vi "Removable devices detection v8.5.vi"() -> (0 "Drive Number":i32, 1 "Drives":string[](array[string]), 2 "Drives Types":T1(array[ring]), 3 "Removable":bool, 4 "Removable":string[](array[string]))   [LabVIEW 2016, in "斯坦道CODMn.lvlib"]
uses:
  kernel32.dll
panel:
  out "Count":i32
  in  "stop":bool
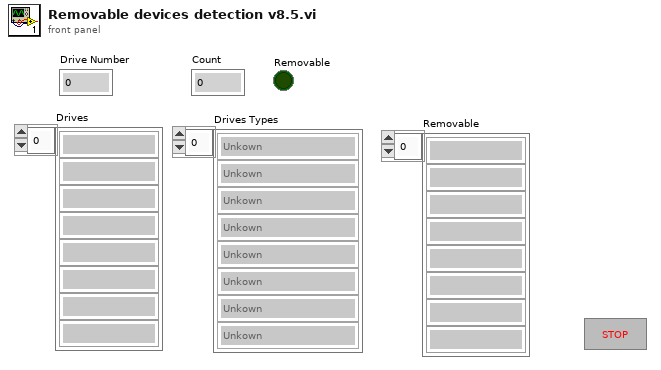
[diagram p1: front panel]
types:
  T1 = enum16{"Unkown", "No Root", "Removable", "Fixed", "Remote Drive", "CD Rom", "Ramdisk"}[]
  T2 = enum16{"Unkown", "No Root", "Removable", "Fixed", "Remote Drive", "CD Rom", "Ramdisk"}
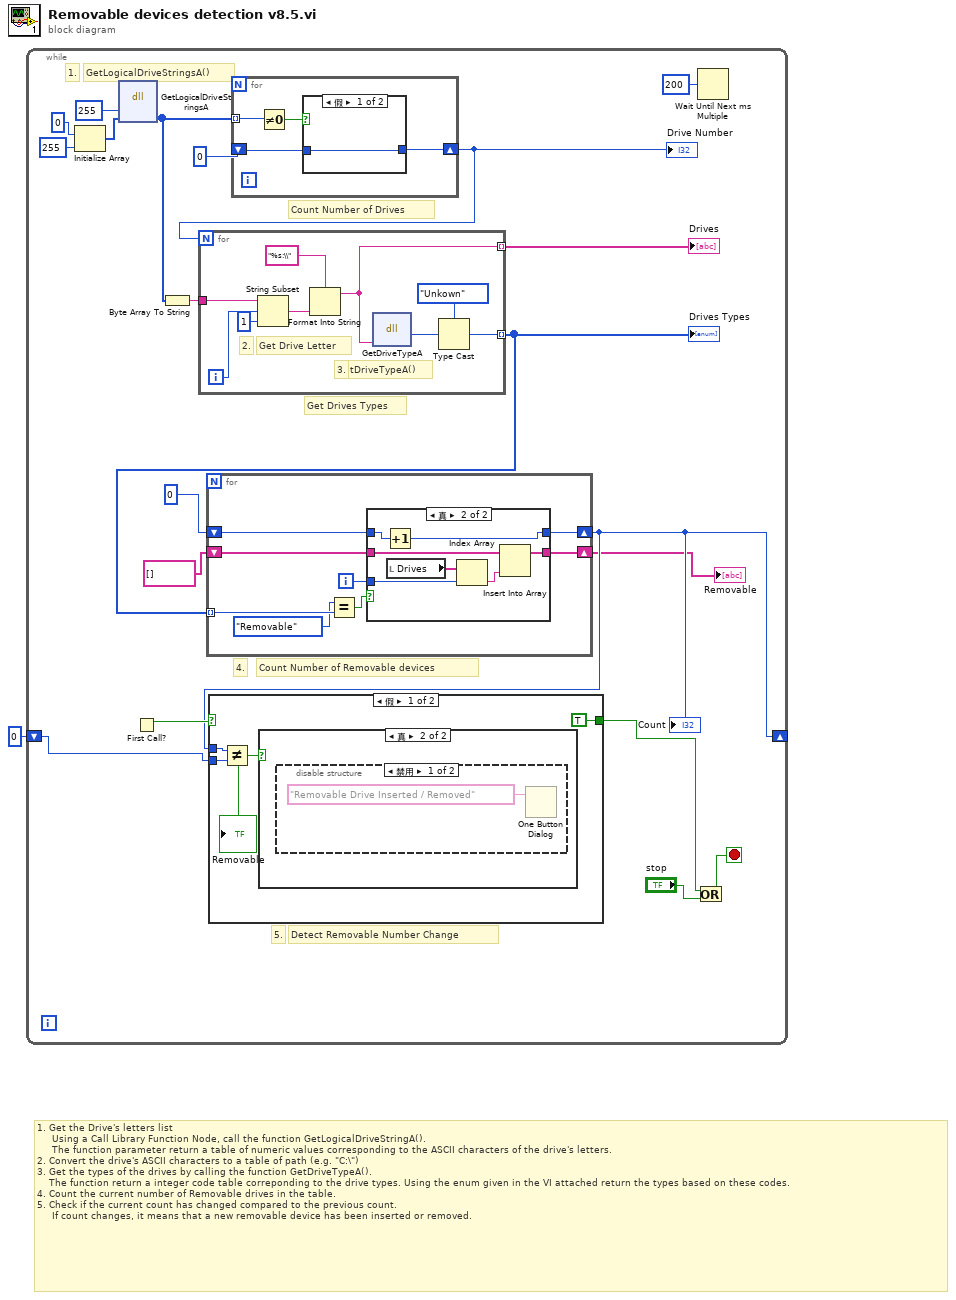
[diagram p0: block diagram]
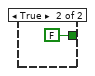
[diagram p4: hidden frame]
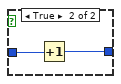
[diagram p6: hidden frame]
diagram:
  # "1. Get the Drive's letters list\n     Using a Call Library Function Node, call the function GetLogicalDriveStringA().\n     The function parameter return a table of numeric values corresponding to the ASCII characters of the drive's letters.\n2. Convert the drive's ASCII characters to a table of path (e.g. \"C:\\\")\n3. Get the types of the drives by calling the function GetDriveTypeA().\n    The function return a integer code table correponding to the drive types. Using the enum given in the VI attached return the types based on these codes.\n4. Count the current number of Removable drives in the table.\n5. Check if the current count has changed compared to the previous count.\n     If count changes, it means that a new removable device has been inserted or removed."
  n1 = while {
    shift-right: [w8] -> _
    shift-left: 0 -> [w9]
    stop <- w2 stop-if-true
    # "5."
    # "4."
    # "1."
    # "Count Number of Drives"
    # "Get Drives Types"
    # "Count Number of Removable devices"
    # "Detect Removable Number Change"
    # "GetLogicalDriveStringsA()"
    n2 = Initialize Array(0 ("arg1"), 255 ("taille de la dimension")) -> (w18:i32[])
    n3 = dll-call lib="kernel32.dll" fn="GetLogicalDriveStringsA"("arg1"=255, "arg2"=w18) -> ("arg2"=w15:i32[])  [unwired: 4 in, 3 out]
    n4 = First Call?() -> (First Call?: T/F=w10:bool)
    n5 = Byte Array To String(unsigned byte array=w15) -> (string=w13:string)
    n6 = for {
      tunnel: w15 -> [w55] mode=indexing
      shift-right: [w56] -> w14
      shift-left: 0 -> [w57]
      n7 = Not Equal To 0?(x=w55) -> (x != 0?=w54:bool)
      n8 = case shown="假" w54 {
        tunnel: w57 -> [w58 w59]
        tunnel: [w58 w60] -> w56
        frame False {
        }
        frame True {
          n9 = Increment(x=w59) -> (x+1=w60:i32)
        }
      }
    }
    "Drive Number" <- w14
    n10 = for {
      N: w14 -> [_]
      tunnel: w13 -> [w50]
      tunnel: [w47] -> w12 mode=indexing
      tunnel: [w46] -> w7 mode=indexing
      i -> [w49]
      # "3."
      # "2."
      # "GetDriveTypeA()"
      # "Get Drive Letter"
      n11 = String Subset(string=w50, offset (0)=w49, length (rest)=1 ("longueur (reste)")) -> (substring=w51:string)
      n12 = Format Into String(format string="%s:\\", w51) -> (resulting string=w47:string)  [unwired: 2 in, 1 out]
      n13 = dll-call lib="kernel32.dll" fn="GetDriveTypeA"("lpRootPathName"=w47) -> ("type de retour"=w45:u16)  [unwired: 3 in, 3 out]
      n14 = Type Cast(type=T2."Unkown" ("Drive Type"), x=w45) -> (*(type *) &x=w46:T2)
    }
    "Drives" <- w12
    "Drives Types" <- w7
    n15 = for {
      tunnel: w7 -> [w35] mode=indexing
      shift-right: [w31] -> w8
      shift-left: 0 -> [w32]
      shift-right: [w28] -> w6
      shift-left: string[] [] -> [w29]
      i -> [w30]
      n16 = Equal?(x=T2."Removable" ("Drive Type"), y=w35) -> (x = y?=w33:bool)
      n17 = case shown="真" w33 {
        tunnel: w32 -> [w37 w44]
        tunnel: [w37 w43] -> w31
        tunnel: w30 -> [_ w41]
        tunnel: w29 -> [w36 w40]
        tunnel: [w36 w39] -> w28
        frame False {
        }
        frame True {
          n18 = Increment(x=w44) -> (x+1=w43:i32)
          n19 = local read "Drives"() -> (w42:string[])
          n20 = Index Array(array=w42, index=w41) -> (element=w38:string)
          n21 = Insert Into Array(array=w40, new element=w38) -> (w39:string[])  [unwired: 1 in]
        }
      }
    }
    "Count" <- w8
    "Removable" <- w6
    n22 = case shown="假" w10 {
      tunnel: w9 -> [w24 _]
      tunnel: w8 -> [w25 _]
      tunnel: [TRUE FALSE] -> w3
      frame False {
        n23 = Not Equal?(x=w25, y=w24) -> (x != y?=w23:bool)
        "Removable" <- w23
        n24 = case shown="真" w23 {
          frame False {
          }
          frame True {
            n25 = disable-structure shown="禁用" {
              frame Disabled {
                n26 = One Button Dialog(message="Removable Drive Inserted / Removed") -> ()  [unwired: 2 out]
              }
              frame Enabled {
              }
            }
          }
        }
      }
      frame True {
      }
    }
    n27 = Or(x=w3, y="stop") -> (x .or. y?=w2:bool)
    n28 = Wait Until Next ms Multiple(millisecond multiple=u32 200 ("n millisecondes")) -> ()  [unwired: 1 out]
  }
